vi "Image Display Rectange ROI Zoom.vi"(8 "Error In":errorcluster, 9 "ROI Descriptor":T1 {"Contours"."Type" items=["No Selection", "Point", "Line", "Rectangle", "Oval", "Polygon", "Freehand Region", "Annulus", "Unused2", "Unused3", "Broken Line", "Freehand Line", "Rotated Rectangle"]}, 11 "Display Image Control Refnum":T2) -> (0 "Error Out":errorcluster)   [LabVIEW 2021, in "Image.lvlib"]
uses:
  Image.lvlib
  Image Control Refnum.ctl
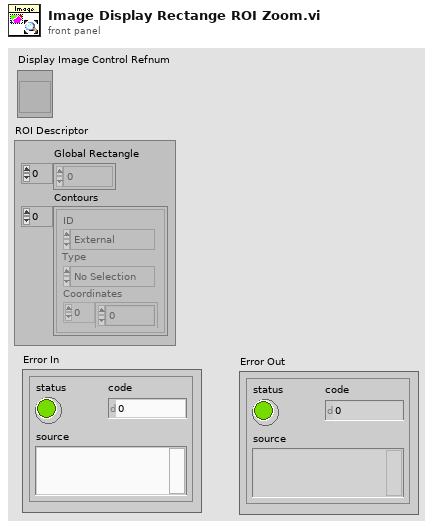
[diagram p1: front panel]
types:
  T1 = typedef "ROI Descriptor" = cluster{"Global Rectangle":i32[], "Contours":cluster{"ID":enum32{"External", "Internal"}, "Type":u32, "Coordinates":i32[]}[]}
  T2 = typedef "Image.lvlib/Image Control Refnum.ctl" = refnum<vi>
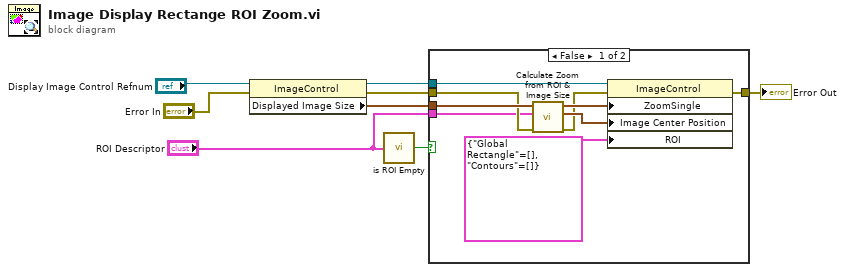
[diagram p0: block diagram]
diagram:
  n1 = property class="ImageControl"(reference="Display Image Control Refnum", error in="Error In") -> (reference out=w5:T2, error out=w3:errorcluster, "Displayed Image Size"=w6:cluster{"Width":u32, "Height":u32})
  n2 = call "is ROI Empty.vi"("Current ROI Descriptor"="ROI Descriptor") -> ("Empty ROI?"=w2:bool)  [unwired: 8 in]
  n3 = case shown="False" w2 {
    tunnel: w6 -> [w17 _]
    tunnel: w5 -> [w16 _]
    tunnel: [w13 w18] -> w4
    tunnel: w3 -> [w11 w18]
    tunnel: "ROI Descriptor" -> [w10 _]
    frame False {
      n4 = call "Calculate Zoom from ROI & Image Size.vi"("Error In"=w11, "ROI Descriptor"=w10, "Displayed Image:Size"=w17) -> ("Error Out"=w12:errorcluster, "Center Position"=w14:cluster{dbl, dbl}, "Zoom Factor"=w15:cluster{dbl, dbl})  [unwired: 6 in]
      n5 = property class="ImageControl"(reference=w16, error in=w12, "ZoomSingle"=w15, "Image Center Position"=w14, "ROI"=T1 {"Global Rectangle"=[], "Contours"=[]} ("ROI Descriptor")) -> (error out=w13:errorcluster)  [unwired: 1 out]
    }
    frame True {
    }
  }
  "Error Out" <- w4
